vi "Report Core.vi"(8 "error in":errorcluster, 9 "Received":path, 10 "Approved":path, 11 "Reporter in":refnum<class "Reporter.lvclass">) -> (0 "error out":errorcluster, 2 "Worked?":bool, 3 "Reporter out":refnum<class "Reporter.lvclass">)   [LabVIEW 2020, in "Approval Tests.lvlib" / "Reporter.lvclass"]
uses:
  Reporter.lvclass
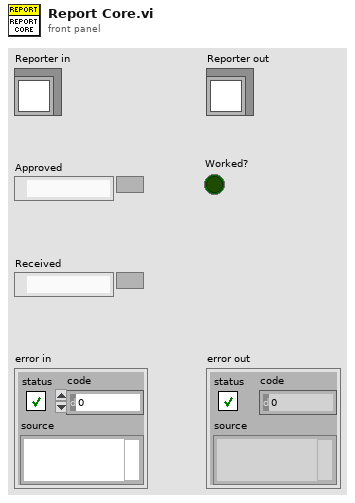
[diagram p1: front panel]
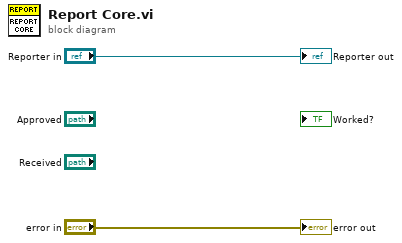
[diagram p0: block diagram]
diagram:
  "error out" <- "error in"
  "Reporter out" <- "Reporter in"
